vi "Send Show GUI Message.vi"(6 "Show GUI Options":T1, 7 "High Priority (F)":bool, 8 "error in (no error)":errorcluster, 11 "MessageQ":refnum<class "MessageQ.lvclass">) -> (0 "error out":errorcluster)   [LabVIEW 2020, in "Volatus.lvlib"]
uses:
  Volatus.lvlib
  MessageQ/MessageQ.lvclass
  MessageQ/MessageQ.lvclass/MessageQ.ctl
  Show GUI Options.ctl
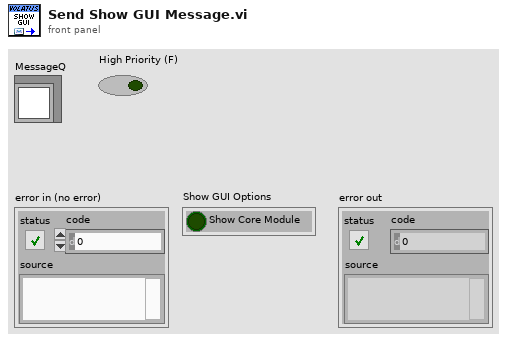
[diagram p1: front panel]
types:
  T1 = typedef "Volatus.lvlib/Show GUI Options.ctl" = cluster{"Show Core Module":bool}
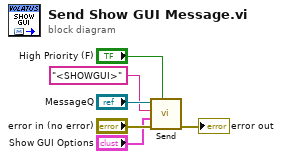
[diagram p0: block diagram]
diagram:
  n1 = call "Send.vi"("High Priority (F)"="High Priority (F)", "error in (no error)"="error in (no error)", "Data"="Show GUI Options", "ID"="<SHOWGUI>", "MessageQ in"="MessageQ") -> ("error out"=→"error out":errorcluster)  [unwired: 5 in, 1 out]
